vi "Read Not_.vi"(8 "error in (no error)":errorcluster, 11 "AssertEqualType in":refnum<class "AssertEqualType.lvclass">) -> (0 "error out":errorcluster, 2 "Not?":bool, 3 "AssertEqualType out":refnum<class "AssertEqualType.lvclass">)   [LabVIEW 2021, in "Bananas.lvlib" / "AssertEqualType.lvclass"]
uses:
  AssertEqualType.lvclass
  AssertEqualType.lvclass/AssertEqualType.ctl
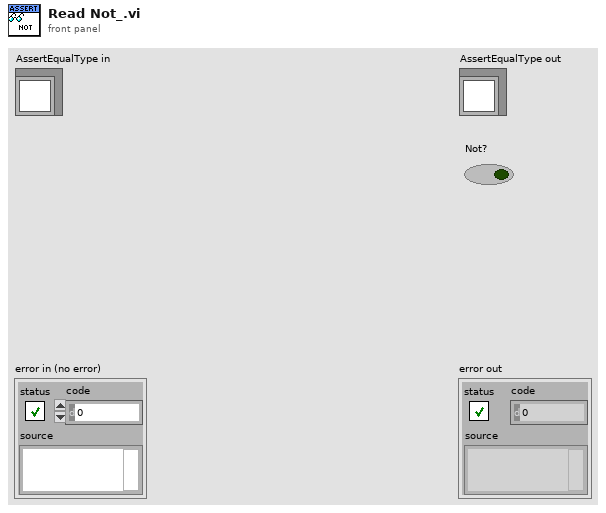
[diagram p1: front panel]
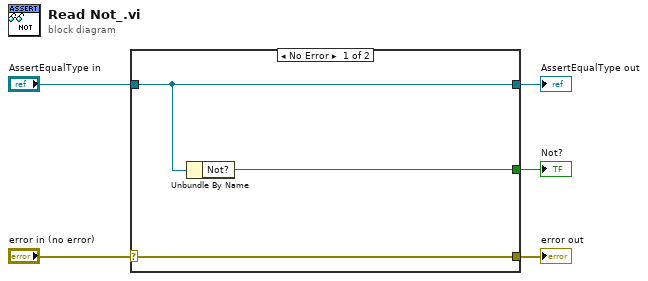
[diagram p0: block diagram]
diagram:
  n1 = case shown="No Error" "error in (no error)" {
    selector: "error in (no error)" -> [w8 w9]
    tunnel: [w8 w9] -> w4
    tunnel: [w7 w10] -> w2
    tunnel: "AssertEqualType in" -> [w7 w10]
    tunnel: [w6 _] -> w1
    frame No Error {
      n2 = Unbundle By Name(w7) -> ("Not?"=w6:bool)
    }
    frame Error {
    }
  }
  "error out" <- w4
  "AssertEqualType out" <- w2
  "Not?" <- w1
